vi "HitrapGUI.StepMotorActivity.vi"(0 "i ref in":refnum<vi>, 1 "DIMPositioncontrolRef":refnum<vi>, 2 "Data":variant, 5 "error in":errorcluster) -> (14 "i ref out":refnum<vi>, 15 "MotorName":string, 16 "StartPosition":i32, 17 "StopPosition":i32, 19 "error out":errorcluster)   [LabVIEW 2014, in "HitrapGUI.lvlib"]
uses:
  HitrapGUI.lvlib
  CS_Core/CSSystem/CoreDefs/CoreDefs.rawDataType.ctl
  CSlibraries-extern/DimLVEvent/LVDimInterface/LVDimInterface.lvlib
  CS_Core/BaseProcess/BaseProcess.lvlib
  CSlibraries-extern/DimLVEvent/DimIndicators/DimIndicators.lvlib
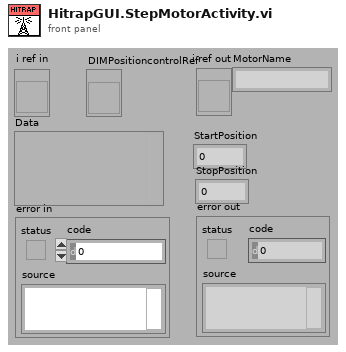
[diagram p1: front panel]
types:
  T1 = typedef "CoreDefs.rawDataType.ctl" = i8[]
  T2 = cluster{"ControlRef":refnum<vi>, "NewPosition2Nom":T1}
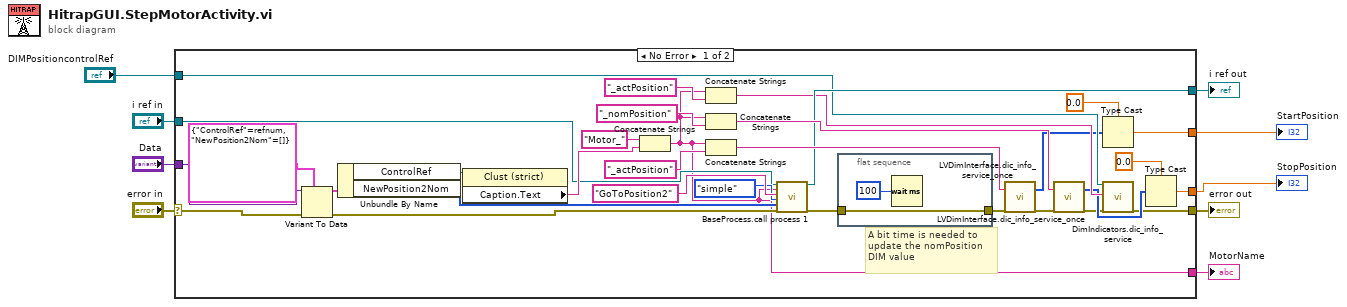
[diagram p0: block diagram]
diagram:
  n1 = case shown="No Error" "error in" {
    selector: "error in" -> [w22 w45]
    tunnel: "i ref in" -> [w29 w44]
    tunnel: "Data" -> [w26 _]
    tunnel: [w25 _] -> w7
    tunnel: [w24 _] -> w6
    tunnel: [w10 w45] -> w5
    tunnel: [w21 w44] -> w3
    tunnel: "DIMPositioncontrolRef" -> [w20 _]
    tunnel: [w11 _] -> w1
    frame No Error {
      # "A bit time is needed to\nupdate the nomPosition\nDIM value"
      n2 = Variant To Data(error in=w22, type=T2 {"ControlRef"=refnum, "NewPosition2Nom"=[]} ("output cluster"), Variant=w26) -> (data=w27:T2, error out=w23:errorcluster)
      n3 = Unbundle By Name(w27) -> ("ControlRef"=w33:refnum<vi>, "NewPosition2Nom"=w30:T1)
      n4 = property class="Clust (strict)"(reference=w33) -> ("Caption.Text"=w40:string)  [unwired: 1 in, 2 out]
      n5 = Concatenate Strings("Motor_" ("string"), w40) -> (w11:string)
      n6 = Concatenate Strings(w11, "_actPosition" ("serviceName")) -> (w18:string)
      n7 = Concatenate Strings(w11, "_nomPosition" ("string")) -> (w38:string)
      n8 = Concatenate Strings(w11, "_actPosition" ("string")) -> (w39:string)
      n9 = call "BaseProcess.call process 1.vi"("i ref in"=w29, "Object"=w11, "Selector"="GoToPosition2", "CallType"=enum16{"simple", "synchronous", "asynchronous"}."simple", "Data"=w30, "error in (no error)"=w23) -> ("i ref out"=w21:refnum<vi>, "error out"=w13:errorcluster)  [unwired: 11 in, 1 out]
      n10 = flat-sequence {
        tunnel: w13 -> [w43]
        tunnel: [w43] -> w12
        frame #0 {
          n11 = Wait (ms)(milliseconds to wait=u32 100) -> ()  [unwired: 1 out]
        }
      }
      n12 = call "LVDimInterface.dic_info_service_once.vi"("serviceName"=w39, "error in (no error)"=w12) -> ("data"=w17:i8[], "error out"=w16:errorcluster)  [unwired: 14 in, 2 out]
      n13 = call "LVDimInterface.dic_info_service_once.vi"("serviceName"=w38, "error in (no error)"=w16) -> ("data"=w15:i8[], "error out"=w14:errorcluster)  [unwired: 14 in, 2 out]
      n14 = Type Cast(type=0.0, x=w17) -> (*(type *) &x=w25:dbl)
      n15 = call "DimIndicators.dic_info_service.vi"("controlRef"=w20, "serviceName"=w18, "error in (no error)"=w14) -> ("error out"=w10:errorcluster)  [unwired: 15 in, 1 out]
      n16 = Type Cast(type=0.0, x=w15) -> (*(type *) &x=w24:dbl)
    }
    frame Error {
    }
  }
  "StartPosition" <- w7
  "StopPosition" <- w6
  "error out" <- w5
  "i ref out" <- w3
  "MotorName" <- w1
